vi "Calc Inputs.vi"(8 "error in (no error)":errorcluster, 11 "Max Calc in":refnum<class "Max Calc.lvclass">) -> (0 "error out":errorcluster, 2 "Inputs":string[](array[string]))   [LabVIEW 2020, in "VolatusCalcs.lvlib" / "Max Calc.lvclass"]
uses:
  Max Calc.lvclass
  Max Calc.lvclass/Max Calc.ctl
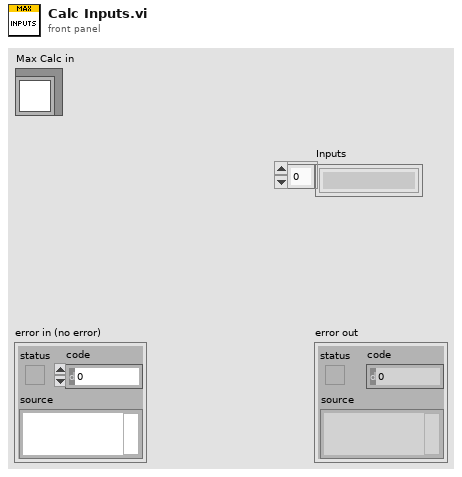
[diagram p1: front panel]
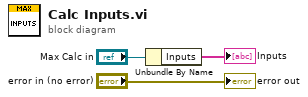
[diagram p0: block diagram]
diagram:
  n1 = Unbundle By Name("Max Calc in") -> ("Inputs"=→"Inputs":string[])
  "error out" <- "error in (no error)"
